vi "ShutdownMode.vi"(8 "error in (no error)":errorcluster, 11 "Watchdog":refnum<data-value>) -> (0 "error out":errorcluster, 3 "Watchdog":refnum<data-value>)   [LabVIEW 2017, in "Watchdog.lvclass"]
doc: "Set the Pound to be in shutdown mode. In shutdown mode, the Pound will check to make sure that each process <b>stops executing</b> within the timeout."
uses:
  <vilib>/NI/Software Watchdog/Watchdog/Watchdog.lvclass
  <vilib>/NI/Software Watchdog/Watchdog/Watchdog.lvclass/Watchdog.ctl
  <vilib>/NI/Software Watchdog/Pound/Write Shutdown Timestamp.vi
  <vilib>/NI/Software Watchdog/Pound/Write Mode.vi
  <vilib>/NI/Software Watchdog/Pound/Pound.lvclass
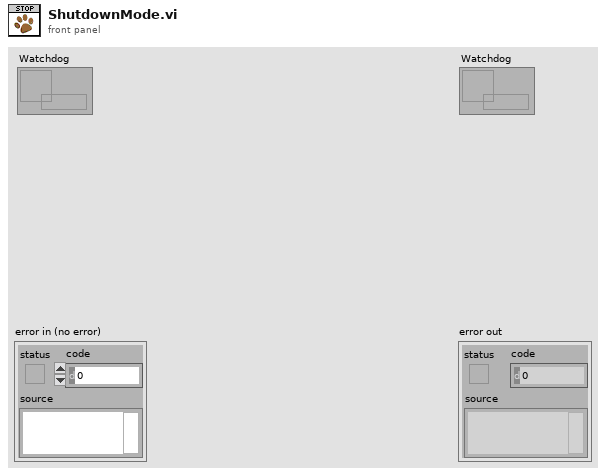
[diagram p1: front panel]
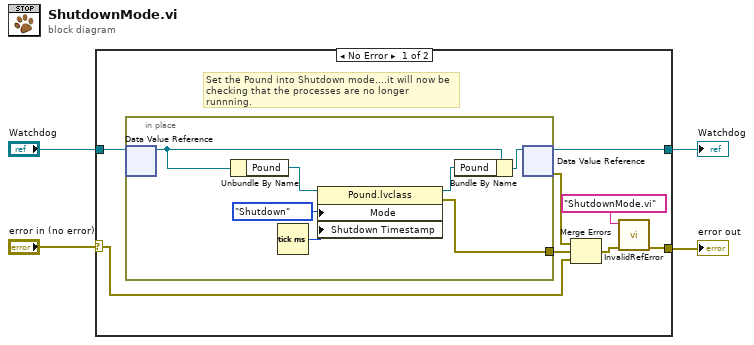
[diagram p0: block diagram]
diagram:
  n1 = case shown="No Error" "error in (no error)" {
    selector: "error in (no error)" -> [w5 w20]
    tunnel: [w7 w20] -> w4
    tunnel: "Watchdog" -> [w12 w21]
    tunnel: [w9 w21] -> w2
    frame No Error {
      # "Set the Pound into Shutdown mode....it will now be checking that the processes are no longer runnning."
      n2 = in-place {
        in-place-border: [w18] -> w11
        n3 = in-place-dvr #1(w12) -> (w15:refnum<class "Watchdog.lvclass">)  [unwired: 1 out]
        n4 = Unbundle By Name(w15) -> ("Pound"=w19:refnum<class "Pound.lvclass">)
        n5 = Tick Count (ms)() -> (millisecond timer value=w16:u32)
        n6 = property class="Pound.lvclass"(reference=w19, "Mode"=enum16{"Running", "Shutdown"}."Shutdown", "Shutdown Timestamp"=w16) -> (reference out=w13:refnum<class "Pound.lvclass">, error out=w18:errorcluster)  [unwired: 1 in]
        n7 = Bundle By Name(cluster=w15, "Pound"=w13) -> (w14:refnum<class "Watchdog.lvclass">)
        n8 = in-place-dvr #1(w14) -> (w9:refnum<data-value>, w10:errorcluster)
      }
      n9 = Merge Errors(w10, w11, w5) -> (w8:errorcluster)
      n10 = call <vilib>:"InvalidRefError.vi"("error in (no error)"=w8, "VI Name"="ShutdownMode.vi") -> ("error out"=w7:errorcluster)  [unwired: 9 in]
    }
    frame Error {
    }
  }
  "error out" <- w4
  "Watchdog" <- w2
